vi "Min Read Array.vi"(8 "error in":errorcluster, 11 "Min Flow Limit in":refnum<class "Flow Limit.lvclass">) -> (0 "error out":errorcluster, 1 "Changed or First Call?":bool, 2 "Flow Min SP":dbl[](array[numeric]), 3 "Min Flow Limit out":refnum<class "Flow Limit.lvclass">)   [LabVIEW 2023, in "Flow Limit.lvclass"]
uses:
  Flow Limit.lvclass
  Flow Limit.lvclass/Flow Limit.ctl
  Parents/Limit/Limit.lvclass
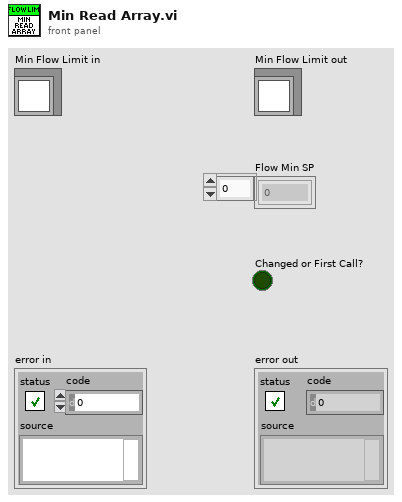
[diagram p1: front panel]
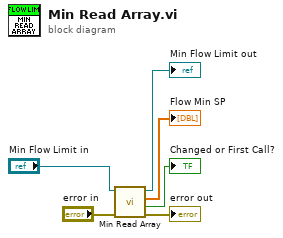
[diagram p0: block diagram]
diagram:
  n1 = call-parent "Min Read Array.vi"("error in"="error in", "Min Limit in"="Min Flow Limit in") -> ("error out"=→"error out":errorcluster, "Changed or First Call?"=→"Changed or First Call?":bool, "Current Min SP"=→"Flow Min SP":dbl[], "Min Limit out"=→"Min Flow Limit out":refnum<class "Flow Limit.lvclass">)  [unwired: 6 in]
